vi "Obtain Task Notifiers and Queues.vi"(8 "error in (no error)":errorcluster, 11 "Task Base in":refnum<class "Task Base.lvclass">) -> (0 "error out":errorcluster, 3 "Task Base out":refnum<class "Task Base.lvclass">)   [LabVIEW 2023, in "HAL GOOP4.lvlib" / "Task Base.lvclass"]
uses:
  Task/Task Base/Task Base.lvclass
  Task/Task Base/Task Base.lvclass/Task Base.ctl
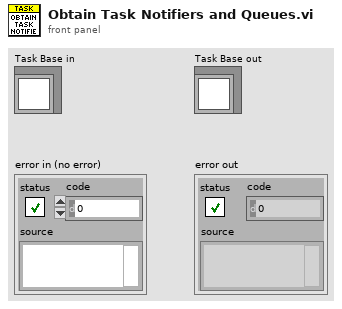
[diagram p1: front panel]
types:
  T1 = cluster{"Stop PE":refnum<notifier>, "Data":refnum<notifier>}
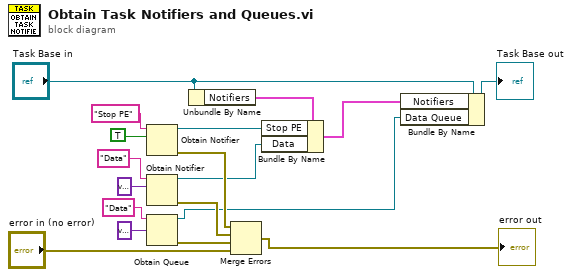
[diagram p0: block diagram]
diagram:
  n1 = Obtain Notifier(name (unnamed)="Stop PE", notification data type=TRUE) -> (notifier out=w7:refnum<notifier>, error out=w11:errorcluster)  [unwired: 2 in, 1 out]
  n2 = Obtain Notifier(name (unnamed)="Data", notification data type=variant) -> (notifier out=w6:refnum<notifier>, error out=w10:errorcluster)  [unwired: 2 in, 1 out]
  n3 = Obtain Queue(name (unnamed)="Data", element data type=variant) -> (queue out=w1:refnum<queue>, error out=w9:errorcluster)  [unwired: 3 in, 1 out]
  n4 = Unbundle By Name("Task Base in") -> ("Notifiers"=w3:T1)
  n5 = Merge Errors(w11, w10, w9, "error in (no error)") -> (→"error out":errorcluster)
  n6 = Bundle By Name(cluster=w3, "Stop PE"=w7, "Data"=w6) -> (w2:T1)
  n7 = Bundle By Name(cluster="Task Base in", "Notifiers"=w2, "Data Queue"=w1) -> (→"Task Base out":refnum<class "Task Base.lvclass">)
